vi "AFM_Driver_Manager.DestroyPublicEvents.vi"(8 "error in (no error)":errorcluster, 11 "AFM_Driver_Manager in":refnum<class "AFM_Driver_Manager.lvclass">) -> (0 "error out":errorcluster, 3 "AFM_Driver_Manager out":refnum<class "AFM_Driver_Manager.lvclass">)   [LabVIEW 2019, in "AFM_Driver_Manager.lvclass"]
uses:
  AFM_Driver_Manager.lvclass
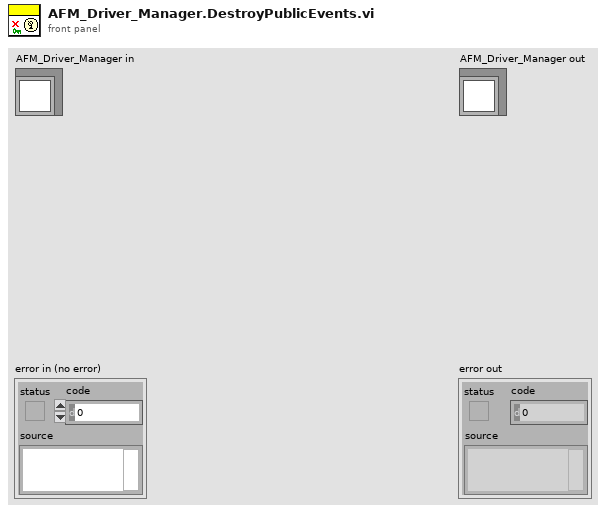
[diagram p1: front panel]
types:
  T1 = typedef "AFM_Driver_Manager.lvclass/AFM_Driver_Manager.PublicEvents.ctl" = cluster{"Lithography Done":refnum<user-event>}
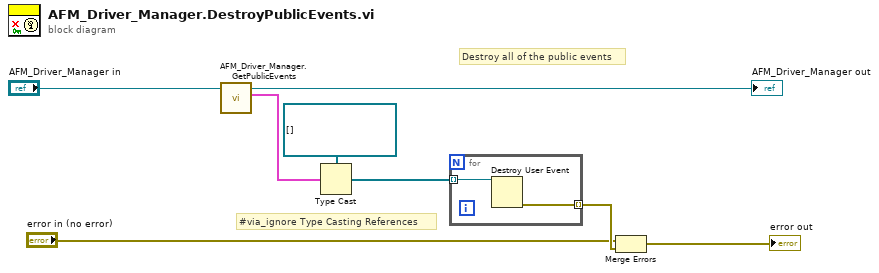
[diagram p0: block diagram]
diagram:
  # "Destroy all of the public events"
  # "#via_ignore Type Casting References"
  n1 = call "AFM_Driver_Manager.GetPublicEvents.vi"("AFM_Driver_Manager in"="AFM_Driver_Manager in") -> ("AFM_Driver Events"=w5:T1, "AFM_Driver_Manager out"=→"AFM_Driver_Manager out":refnum<class "AFM_Driver_Manager.lvclass">)  [unwired: 8 in, 1 out]
  n2 = Type Cast(type=refnum<user-event>[] [], x=w5) -> (*(type *) &x=w4:refnum<user-event>[])
  n3 = for {
    tunnel: w4 -> [w10] mode=indexing
    tunnel: [w9] -> w3 mode=indexing
    n4 = Destroy User Event(user event=w10) -> (error out=w9:errorcluster)  [unwired: 1 in]
  }
  n5 = Merge Errors("error in (no error)", w3) -> (→"error out":errorcluster)
